vi "setSerialSettings.vi"(10 "Serial Settings":T1={"Baud Rate"=921600, "Data Bits"=8, "Parity"=enum."None", "Flow Control"=0, "Stop Bits"=10, "Timeout (ms)"=2000, "Byte Count"=256, "Enable Termination Character"=FALSE, "Termination Char"=200} {"Termination Char" format="%x"; "Stop Bits" items=["1.0"=10, "1.5"=15, "2.0"=20]; "Flow Control" items=["None", "XON/XOFF", "RTS/CTS", "XON/XOFF & RTS/CTS", "DTR/DSR", "XON/XOFF & DTR/DSR"]; "Data Bits" min=5 max=8 step=1}, 11 "DesktopModbus in":refnum<class "DesktopModbus.lvclass">) -> (3 "DesktopModbus out":refnum<class "DesktopModbus.lvclass">)   [LabVIEW 2016, in "DesktopModbus.lvclass"]
uses:
  DesktopModbus.lvclass
  Typedefs/SerialSettings.ctl
  DesktopModbus.lvclass/DesktopModbus.ctl
  Typedefs/HPMT_Typedefs.lvlib
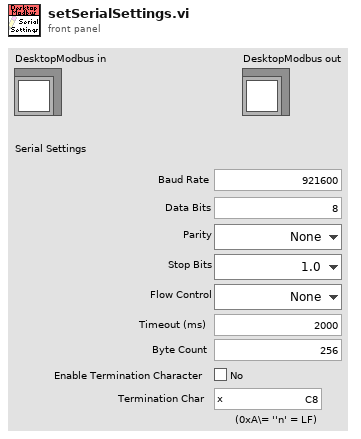
[diagram p1: front panel]
types:
  T1 = typedef "HPMT_Typedefs.lvlib/SerialSettings.ctl" = cluster{"Baud Rate":u32, "Data Bits":u16, "Parity":enum16{"None", "Odd", "Even", "Mark", "Space"}, "Flow Control":u16, "Stop Bits":u16, "Timeout (ms)":u32, "Byte Count":u32, "Enable Termination Character":bool, "Termination Char":u8}
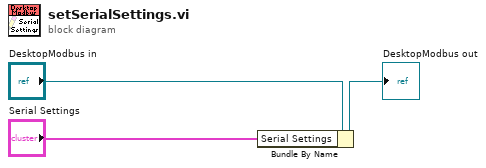
[diagram p0: block diagram]
diagram:
  n1 = Bundle By Name(cluster="DesktopModbus in", "Serial Settings"="Serial Settings") -> (→"DesktopModbus out":refnum<class "DesktopModbus.lvclass">)
